vi "NextStates.vi"(8 "Error In":errorcluster, 10 "States":string[](array[string]), 11 "Queue In":refnum<queue>) -> (0 "Error Out":errorcluster, 3 "Queue Out":refnum<queue>)   [LabVIEW 2010]
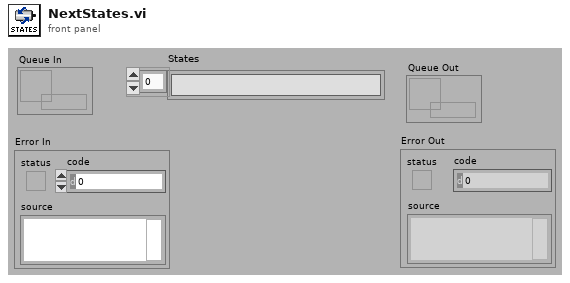
[diagram p1: front panel]
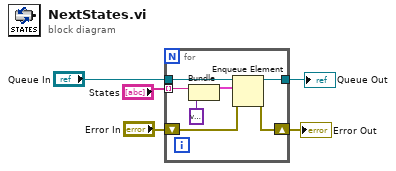
[diagram p0: block diagram]
diagram:
  n1 = for {
    tunnel: "Queue In" -> [w11]
    tunnel: [w10] -> w4
    tunnel: "States" -> [w6] mode=indexing
    shift-right: [w9] -> w3
    shift-left: "Error In" -> [w8]
    n2 = Bundle("State"=w6, "Data"=variant) -> (w12:cluster{"State":string, "Data":variant})  [unwired: 1 in]
    n3 = Enqueue Element(queue=w11, element=w12, error in (no error)=w8) -> (queue out=w10:refnum<queue>, error out=w9:errorcluster)  [unwired: 1 in, 1 out]
  }
  "Queue Out" <- w4
  "Error Out" <- w3
